vi "Core.vi"(0 "Vq":sgl, 1 "registers":T3={"PLLGains"="PLLGains", "PLLRange"="PLLRange", "PLL_reset"="PLL_reset", "PLL_locked"="PLL_locked", "freqBoundaries"="freqBoundaries", "expectedFreq"="expectedFreq", "lockDuration"="lockDuration", "dT"="dT", "detectedFreq"="detectedFreq", "adjustTheta"="adjustTheta", "HarmonicFilter"="HarmonicFilter", "HarmonicFilterEnable"="HarmonicFilterEnable"}, 11 "ThetaIn":sgl, 12 "StateIn":T2) -> (4 "gridFrequency":sgl, 6 "Locked":bool, 10 "adjustedTheta":sgl, 14 "StateOut":T2, 15 "ThetaOut":sgl)   [LabVIEW 2017, in "ThreePhasePLL.lvlib"]
uses:
  ThreePhasePLL.lvlib
  registers.ctl
  <vilib>/rvi/Analysis/control/PID/Typedef/niFpgaPID_PIState.ctl
  <vilib>/rvi/DataTransferAndStorage/Container/Common/niFpgaContainerExecOnDevCompGetState.vi
  <vilib>/rvi/Emulation/niFpgaEmulationIsFPGAContextNoSignature.vi
  <vilib>/rvi/DataTransferAndStorage/Container/Common/niFpgaContainerGetUniqueNameForEmu.vi
  <vilib>/rvi/Memory/Memory_Emulation/niFpgaMemoryEmulationCacheClearOnFirstRun.vi
  <vilib>/rvi/Memory/Memory_Emulation/nirvimemoryEmulationManagerCache_MakeExclusive.vi
  <vilib>/rvi/Memory/Memory_Emulation/niFpgaMemoryEmulationValidateCache.vi
  <vilib>/rvi/Memory/Memory_Emulation/nirvimemoryEmulationManagerCache_InsertValue.vi
  <vilib>/Utility/error.llb/Clear Errors.vi
  <vilib>/rvi/Memory/Memory_Emulation/nirvimemoryEmulationManagerCache_ReleaseExclusive.vi
  <vilib>/rvi/Memory/Memory_Emulation/nirvimemoryEmulationManagerCache_GetValue.vi
  <vilib>/rvi/Memory/Memory_Emulation/nirvimemoryEmulationManagerCache_SetValue.vi
  <vilib>/rvi/Emulation/niFpgaProcessEmulError.vi
  <vilib>/rvi/Emulation/niFpgaSctlEmulationGetInTimedLoop.vi
  <userlib>/_NI FLP Library/addons/Filter/IIRDirectFormIITrans1stOrder/FlpLib IIRDirectFormIITrans1stOrder 0.vi
  <userlib>/_NI FLP Library/FPGA/outsideSCTL/FlpLib Subtract Shared Instance 0.vi
  <userlib>/_NI FLP Library/FPGA/outsideSCTL/FlpLib Add Shared Instance 0.vi
  <userlib>/_NI FLP Library/addons/PowerElectronics/ThreePhasePLL/FlpLib ThreePhasePLL 0.vi
  <userlib>/_NI FLP Library/FPGA/outsideSCTL/FlpLib In Range and Coerce Shared Instance 0.vi
  <vilib>/rvi/DataTransferAndStorage/Container/XNode/niFpgaContainer.xnode
  <vilib>/rvi/DataTransferAndStorage/Register/Emulation/niFpgaRegisterEmulationRefIn.vi
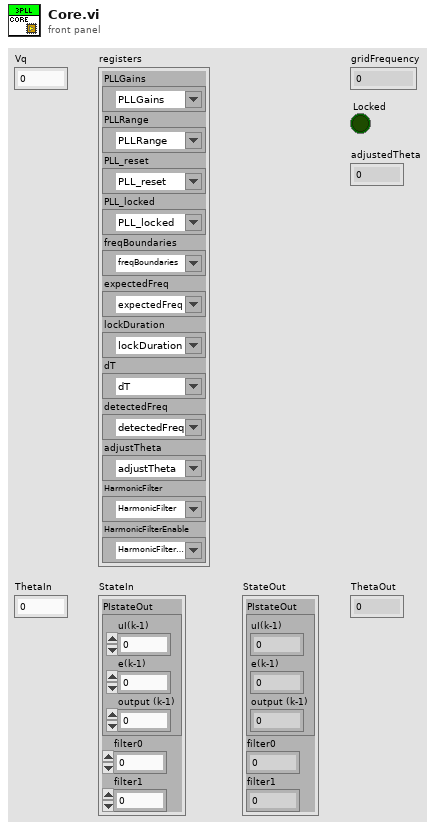
[diagram p1: front panel]
types:
  T1 = typedef "niFpgaPID_PIState.ctl" = cluster{"uI(k-1)":sgl, "e(k-1)":sgl, "output (k-1)":sgl}
  T2 = cluster{"PIstateOut":T1, "filter0":sgl, "filter1":sgl}
  T3 = typedef "ThreePhasePLL.lvlib/registers.ctl" = cluster{"PLLGains":refnum<k21>, "PLLRange":refnum<k21>, "PLL_reset":refnum<k21>, "PLL_locked":refnum<k21>, "freqBoundaries":refnum<k21>, "expectedFreq":refnum<k21>, "lockDuration":refnum<k21>, "dT":refnum<k21>, "detectedFreq":refnum<k21>, "adjustTheta":refnum<k21>, "HarmonicFilter":refnum<k21>, "HarmonicFilterEnable":refnum<k21>}
  T4 = cluster{"output high (Inf)":sgl, "output low (-Inf)":sgl}
  T5 = cluster{"proportional gain":sgl, "integral gain":sgl}
  T6 = cluster{"PIstateOut":T1, "stateOut":sgl, "stateOut":sgl}
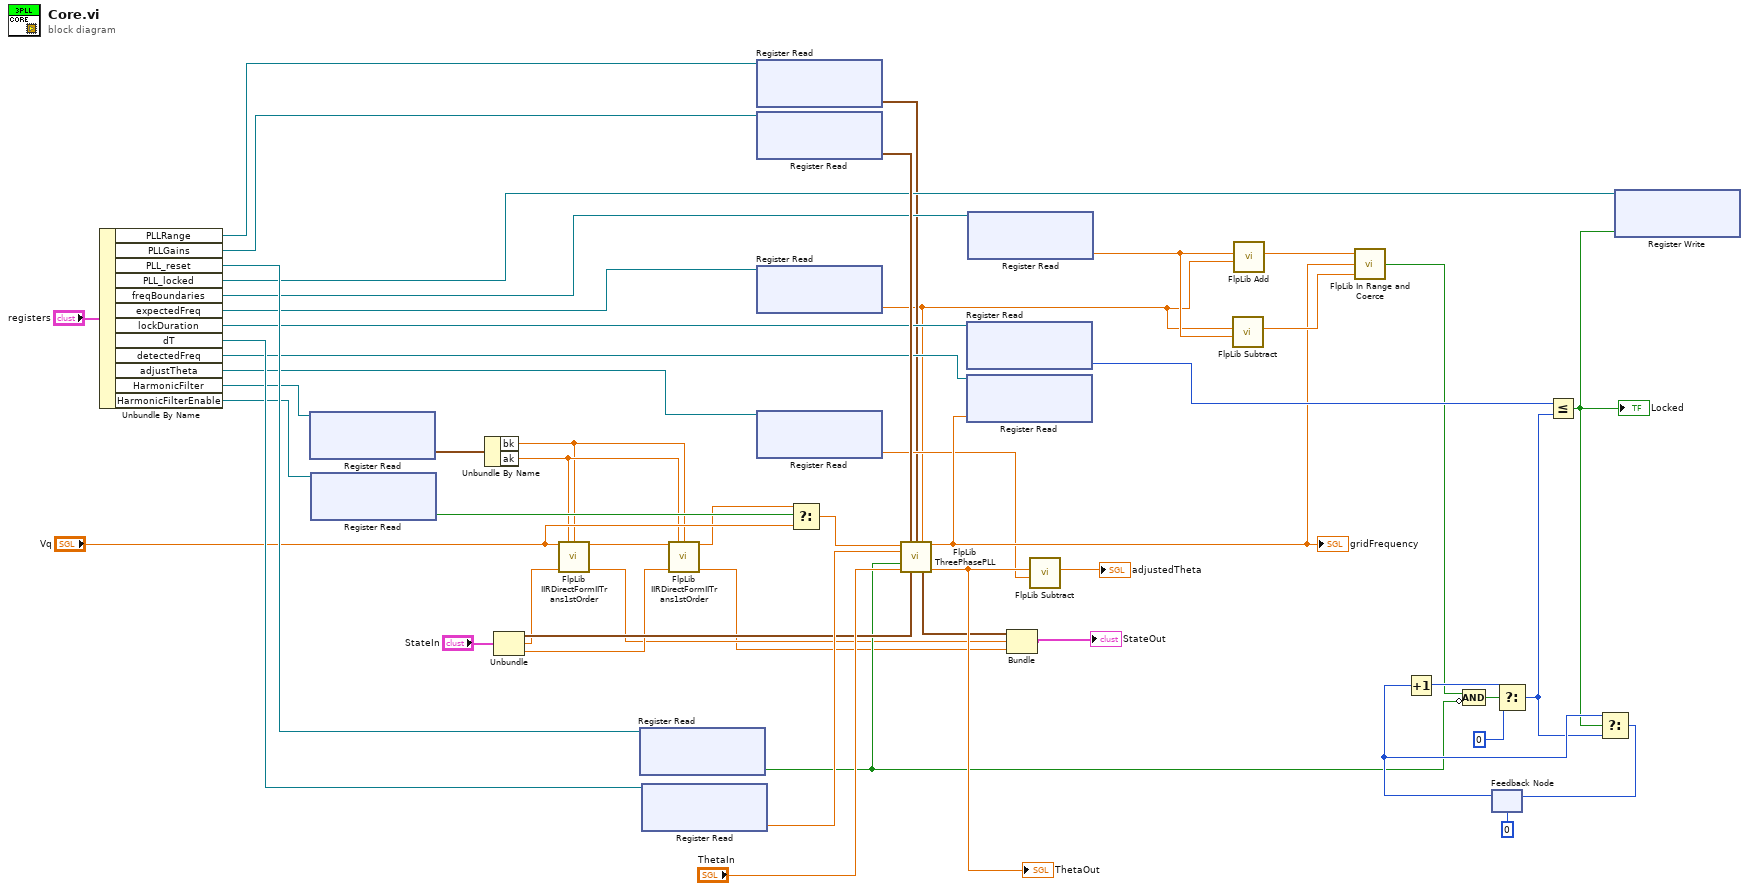
[diagram p0: block diagram]
diagram:
  n1 = Unbundle By Name("registers") -> ("PLLRange"=w47:refnum<k21>, "PLLGains"=w51:refnum<k21>, "PLL_reset"=w46:refnum<k21>, "PLL_locked"=w34:refnum<k21>, "freqBoundaries"=w44:refnum<k21>, "expectedFreq"=w45:refnum<k21>, "lockDuration"=w40:refnum<k21>, "dT"=w49:refnum<k21>, "detectedFreq"=w29:refnum<k21>, "adjustTheta"=w27:refnum<k21>, "HarmonicFilter"=w21:refnum<k21>, "HarmonicFilterEnable"=w19:refnum<k21>)
  n2 = xnode ("Register Read")("Register In"=w21) -> ("Data"=w20:cluster{"ak":sgl, "bk":sgl})  [unwired: 1 out]
  n3 = xnode ("Register Read")("Register In"=w19) -> ("Data"=w18:bool)  [unwired: 1 out]
  n4 = Unbundle By Name(w20) -> ("bk"=w5:sgl, "ak"=w6:sgl)
  n5 = Unbundle("StateIn") -> ("PIstateOut"=w11:T1, "filter0"=w10:sgl, "filter1"=w4:sgl)
  n6 = call-poly <userlib>:"FlpLib IIRDirectFormIITrans1stOrder.vi"("xn"="Vq", "ak"=w6, "bk"=w5, "stateIn"=w10) -> ("yn"=w8:sgl, "stateOut"=w2:sgl)  [unwired: 10 in]
  n7 = xnode ("Register Read")("Register In"=w46) -> ("Data"=w9:bool)  [unwired: 1 out]
  n8 = xnode ("Register Read")("Register In"=w49) -> ("Data"=w48:sgl)  [unwired: 1 out]
  n9 = call-poly <userlib>:"FlpLib IIRDirectFormIITrans1stOrder.vi"("xn"=w8, "ak"=w6, "bk"=w5, "stateIn"=w4) -> ("yn"=w7:sgl, "stateOut"=w1:sgl)  [unwired: 10 in]
  n10 = xnode ("Register Read")("Register In"=w47) -> ("Data"=w15:T4)  [unwired: 1 out]
  n11 = xnode ("Register Read")("Register In"=w51) -> ("Data"=w50:T5)  [unwired: 1 out]
  n12 = xnode ("Register Read")("Register In"=w45) -> ("Data"=w14:sgl)  [unwired: 1 out]
  n13 = xnode ("Register Read")("Register In"=w27) -> ("Data"=w25:sgl)  [unwired: 1 out]
  n14 = Select(t=w7, s=w18, f="Vq") -> (s? t:f=w16:sgl)
  n15 = call-poly <userlib>:"FlpLib ThreePhasePLL.vi"("Vq"=w16, "PLLgains"=w50, "PLLrange"=w15, "expectedFreq"=w14, "dT"=w48, "reset"=w9, "Phase In"="ThetaIn", "PIstateIn"=w11) -> ("gridFrequency"=w28:sgl, "PIstateOut"=w13:T1, "Phase Out"=w26:sgl)  [unwired: 5 in]
  "ThetaOut" <- w26
  "gridFrequency" <- w28
  n16 = xnode ("Register Read")("Register In"=w40) -> ("Data"=w31:u32)  [unwired: 1 out]
  n17 = xnode ("Register Read")("Data"=w28, "Register In"=w29) -> ()  [unwired: 1 out]
  n18 = xnode ("Register Read")("Register In"=w44) -> ("Data"=w43:sgl)  [unwired: 1 out]
  n19 = Bundle("PIstateOut"=w13, "stateOut"=w2, "stateOut"=w1) -> (→"StateOut":T6)  [unwired: 1 in]
  n20 = call-poly <userlib>:"FlpLib Subtract.vi"("y"=w25, "x"=w26) -> ("x-y"=→"adjustedTheta":sgl)  [unwired: 5 in]
  n21 = call-poly <userlib>:"FlpLib Subtract.vi"("y"=w43, "x"=w14) -> ("x-y"=w41:sgl)  [unwired: 5 in]
  n22 = call-poly <userlib>:"FlpLib Add.vi"("y"=w14, "x"=w43) -> ("x+y"=w42:sgl)  [unwired: 5 in]
  n23 = call-poly <userlib>:"FlpLib In Range and Coerce.vi"("lower limit"=w41, "x"=w28, "upper limit"=w42) -> ("in range?"=w23:bool)  [unwired: 1 in, 1 out]
  n24 = Compound Arithmetic op=AND(w23, invert w9) -> (w22:bool)
  n25 = feedback #1(u32 0 ("Data")) -> (w35:u32)
  n26 = Increment(x=w35) -> (x+1=w37:u32)
  n27 = Select(t=w37, s=w22, f=u32 0 ("Data")) -> (s? t:f=w30:u32)
  n28 = Less Or Equal?(x=w31, y=w30) -> (x <= y?=w33:bool)
  "Locked" <- w33
  n29 = Select(t=w35, s=w33, f=w30) -> (s? t:f=w36:u32)
  n30 = feedback-in #1(w36) -> ()
  n31 = xnode ("Register Write")("Data"=w33, "Register In"=w34) -> ()  [unwired: 1 out]
